vi "convert to seconds.vi"(7 "interval scale (s)":T1=enum."s", 11 "Value in":dbl) -> (2 "ms out":dbl, 3 "seconds out":dbl)   [LabVIEW 2023]
doc: "converts ms or min values to seconds (given input type, with default to seconds).\n\nNote, months assumes a 30 day month, and is not 100% accurate as a result.\nYears assumes a 365-day year, plus one day for every 4 years, and does not account for additional leap values."
uses:
  interval type.ctl
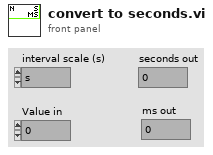
[diagram p1: front panel]
types:
  T1 = typedef "interval type.ctl" = enum16{"ms", "s", "min", "hours", "days", "weeks", "months", "years"}
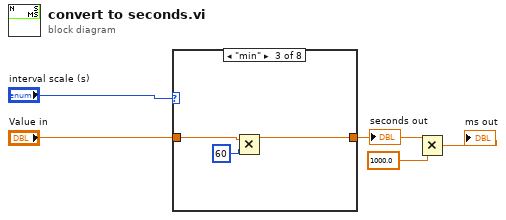
[diagram p0: block diagram]
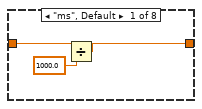
[diagram p2: hidden frame]
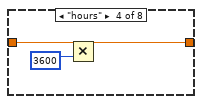
[diagram p4: hidden frame]
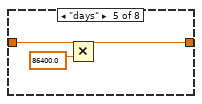
[diagram p5: hidden frame]
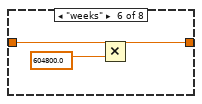
[diagram p6: hidden frame]
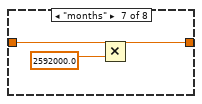
[diagram p7: hidden frame]
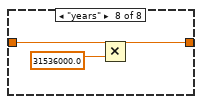
[diagram p8: hidden frame]
diagram:
  n1 = case shown="\"min\"" "interval scale (s)" {
    tunnel: "Value in" -> [w8 w9 w12 w14 w17 w20 w23 w26]
    tunnel: [w6 w9 w10 w13 w16 w19 w22 w25] -> w3
    frame "ms", Default {
      n2 = Divide(x=w8, y=1000.0) -> (x/y=w6:dbl)
    }
    frame "s" {
    }
    frame "min" {
      n3 = Multiply(x=w12, y=60) -> (x*y=w10:dbl)
    }
    frame "hours" {
      n4 = Multiply(x=w14, y=3600) -> (x*y=w13:dbl)
    }
    frame "days" {
      n5 = Multiply(x=w17, y=86400.0) -> (x*y=w16:dbl)
    }
    frame "weeks" {
      n6 = Multiply(x=w20, y=604800.0) -> (x*y=w19:dbl)
    }
    frame "months" {
      n7 = Multiply(x=w23, y=2592000.0) -> (x*y=w22:dbl)
    }
    frame "years" {
      n8 = Multiply(x=w26, y=31536000.0) -> (x*y=w25:dbl)
    }
  }
  "seconds out" <- w3
  n9 = Multiply(x=w3, y=1000.0) -> (x*y=→"ms out":dbl)
